vi "TCRL Host Main.vi"() -> ()   [LabVIEW 2013]
doc: "This application launches and executes the Tag Bus Data framework configuration for the specified target alias. This is a simple example of the framework API functions, but may also be a suitable starting point for a Host UI or Thick Client that is running a local version of the framework."
uses:
  <vilib>/NI/Module Execution Interface/Engine Runtime/Execution States.ctl
  <vilib>/NI/Module Execution Interface/Engine Runtime/Fault.ctl
  <vilib>/NI/Tag Bus Module Framework/runtime/error classification.ctl
  <vilib>/NI/Module Execution Interface/Engine Runtime/Engine Runtime Interface.lvclass
  <vilib>/userdefined/High Color/nirio_resource_hc.ctl
  <vilib>/NI/Tag Bus Data Framework/Framework Configuration Classes/target runtime/PL_Target Runtime.lvclass
  <vilib>/NI/Tag Bus Module Framework/FPGA manager/FPGA manager.lvlib
  <vilib>/rvi/interface/nirviOpenFPGA/nirviOpenFPGA.xnode
  <vilib>/NI/Tag Bus Module Framework/FPGA manager/methods.ctl
  <vilib>/NI/Tag Bus Module Framework/runtime/TBM module execution interface.lvclass
panel:
  in  "configuration file path":path=path "C:/Users/lucamach/Documents/SE/Tagbus/DCAF HO 2016 v2/Excercise 1/RT Temperature Controller - Test 2/SimulatedSystem.pcfg"
  in  "target alias":string="PC"
  out "engine status":T4(array[cluster])
  in  "stop":bool
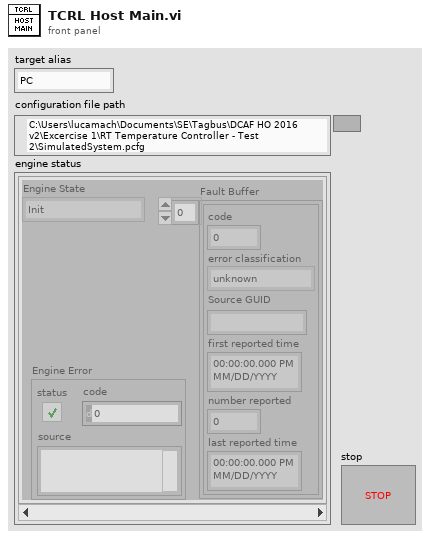
[diagram p1: front panel]
types:
  T1 = typedef "Engine Runtime Interface.lvclass/Execution States.ctl" = enum16{"Init", "Pre-Operational", "Safe-Operational", "Operational", "Stopped"}
  T2 = typedef "Engine Runtime Interface.lvclass/Fault.ctl" = cluster{"code":i32, "error classification":T3, "Source GUID":string, "first reported time":timestamp, "number reported":u32, "last reported time":timestamp}
  T3 = typedef "TBM module execution interface.lvclass/error classification.ctl" = enum16{"unknown", "none", "trivial", "recoverable", "critical"}
  T4 = cluster{"Engine State":T1, "Fault Buffer":T2[], "Engine Error":errorcluster}[]
  T5 = typedef "FPGA manager.lvlib/methods.ctl" = enum16{"initialize bitfile", "cache bitfile", "locate bitfile", "close bitfile", "clear manager"}
  T6 = typedef "nirio_resource_hc.ctl" = tag
  T7 = cluster{"Engine State":T1, "faults":T2[], "Engine Error":errorcluster}
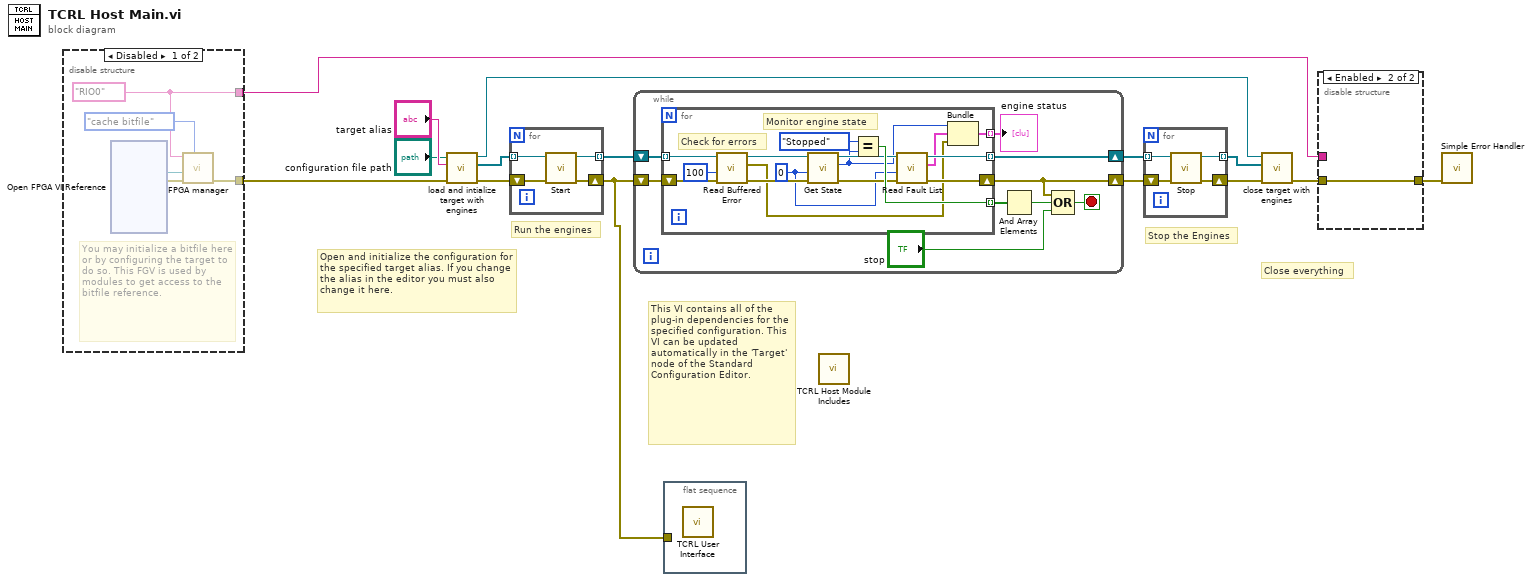
[diagram p0: block diagram]
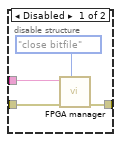
[diagram p2: hidden frame]
diagram:
  # "Open and initialize the configuration for the specified target alias. If you change the alias in the editor you must also change it here."
  # "Close everything"
  # "Stop the Engines"
  # "This VI contains all of the plug-in dependencies for the specified configuration. This VI can be updated automatically in the 'Target' node of the Standard Configuration Editor."
  # "Run the engines"
  n1 = disable-structure shown="Disabled" {
    disable-tunnel: [w20 _] -> w5
    disable-tunnel: [w16 _] -> w2
    frame Disabled {
      w16 = T6 "RIO0" ("RIO resource")
      # "You may initialize a bitfile here or by configuring the target to do so. This FGV is used by modules to get access to the bitfile reference."
      n2 = xnode "Open FPGA VI Reference"() -> ("FPGA VI Reference Out"=w18:refnum<k20>, "error out"=w19:errorcluster)  [unwired: 2 in]
      n3 = call <vilib>:"FPGA manager.vi"("action"=methods."cache bitfile", "error in"=w19, "bitfile to cache"=w18, "RIO resource"=w16) -> ("error out"=w20:errorcluster)  [unwired: 5 in, 2 out]
    }
    frame Enabled {
    }
  }
  n4 = call <vilib>:"load and intialize target with engines.vi"("error in"=w5, "target alias"="target alias", "file path"="configuration file path") -> ("error out"=w12:errorcluster, "engine runtime interfaces"=w11:refnum<class "Engine Runtime Interface.lvclass">[], "target runtime"=w8:refnum<class "PL_Target Runtime.lvclass">)  [unwired: 6 in]
  n5 = for {
    tunnel: [w24] -> w15 mode=indexing
    tunnel: w11 -> [w21] mode=indexing
    shift-right: [w23] -> w1
    shift-left: w12 -> [w22]
    n6 = call-dynamic "Start.vi"("error in"=w22, "Engine Runtime Interface in"=w21) -> ("error out"=w23:errorcluster, "Engine Runtime Interface out"=w24:refnum<class "Engine Runtime Interface.lvclass">)  [unwired: 8 in]
  }
  n7 = while {
    shift-right: [w31] -> w14
    shift-left: w15 -> [w33]
    shift-right: [w28] -> w13
    shift-left: w1 -> [w32]
    stop <- w29 stop-if-true
    n8 = for {
      tunnel: w33 -> [w49] mode=indexing
      tunnel: [w40] -> w31 mode=indexing
      tunnel: [w44] -> w26 mode=indexing
      shift-right: [w39] -> w28
      shift-left: w32 -> [w48]
      tunnel: [w34] -> w27 mode=indexing
      w38 = 0 ("timeout (-1)")
      # "Monitor engine state"
      # "Check for errors"
      n9 = call-dynamic "Read Buffered Error.vi"("error in"=w48, "timeout in ms (0)"=100, "Engine Runtime Interface in"=w49) -> ("error out"=w46:errorcluster, "Engine Error"=w35:errorcluster, "Engine Runtime Interface out"=w47:refnum<class "Engine Runtime Interface.lvclass">)  [unwired: 6 in]
      n10 = call-dynamic "Get State.vi"("error in"=w46, "timeout (-1)"=w38, "Engine Runtime Interface in"=w47) -> ("error out"=w42:errorcluster, "Engine State"=w37:T1, "Engine Runtime Interface out"=w41:refnum<class "Engine Runtime Interface.lvclass">)  [unwired: 6 in]
      n11 = Equal?(x=Execution_States."Stopped" ("Engine State"), y=w37) -> (x = y?=w44:bool)
      n12 = call-dynamic "Read Fault List.vi"("error in"=w42, "timeout (-1)"=w38, "Engine Runtime Interface in"=w41) -> ("error out"=w39:errorcluster, "faults"=w36:T2[], "Engine Runtime Interface out"=w40:refnum<class "Engine Runtime Interface.lvclass">)  [unwired: 6 in]
      n13 = Bundle("Engine State"=w37, "faults"=w36, "Engine Error"=w35) -> (w34:T7)  [unwired: 1 in]
    }
    "engine status" <- w27
    n14 = And Array Elements(Boolean array=w26) -> (logical AND=w25:bool)
    n15 = Compound Arithmetic op=OR(w28, w25, "stop") -> (w29:bool)
  }
  n16 = flat-sequence {
    tunnel: w1 -> [_]
    frame #0 {
      n17 = call "TCRL User Interface.vi"() -> ()  [unwired: 12 in]
    }
  }
  n18 = call "TCRL Host Module Includes.vi"() -> ()  [unwired: 12 in]
  n19 = for {
    tunnel: w14 -> [w53] mode=indexing
    shift-right: [w50] -> w7
    shift-left: w13 -> [w52]
    tunnel: [w51] -> w9 mode=indexing
    n20 = call-dynamic "Stop.vi"("error in"=w52, "Engine Runtime Interface in"=w53) -> ("error out"=w50:errorcluster, "Engine Runtime Interface out"=w51:refnum<class "Engine Runtime Interface.lvclass">)  [unwired: 8 in]
  }
  n21 = call <vilib>:"close target with engines.vi"("error in"=w7, "Engine Runtime Interfaces"=w9, "Target Runtime"=w8) -> ("error out"=w3:errorcluster)  [unwired: 8 in]
  n22 = disable-structure shown="Enabled" {
    disable-tunnel: [w56 w58] -> w4
    disable-tunnel: w3 -> [w57 w58]
    disable-tunnel: w2 -> [w54 _]
    frame Disabled {
      n23 = call <vilib>:"FPGA manager.vi"("action"=methods."close bitfile", "error in"=w57, "RIO resource"=w54) -> ("error out"=w56:errorcluster)  [unwired: 6 in, 2 out]
    }
    frame Enabled {
    }
  }
  n24 = call <vilib>:"Simple Error Handler.vi"("error in (no error)"=w4) -> ()  [unwired: 4 in, 5 out]
